vi "Get Column Headers.vi"(8 "error in (no error)":errorcluster, 11 "Process Tree View in":refnum<class "Process Tree View.lvclass">) -> (0 "error out":errorcluster, 3 "Process Tree View out":refnum<class "Process Tree View.lvclass">)   [LabVIEW 2020, in "Process Tree View.lvclass"]
uses:
  Process Tree View.lvclass
  Process Tree View.lvclass/Process Tree View.ctl
  Process Tree View Model/Process Tree View Model.lvclass
  Tree Helpers/Tag Tree/Tag Tree.lvclass
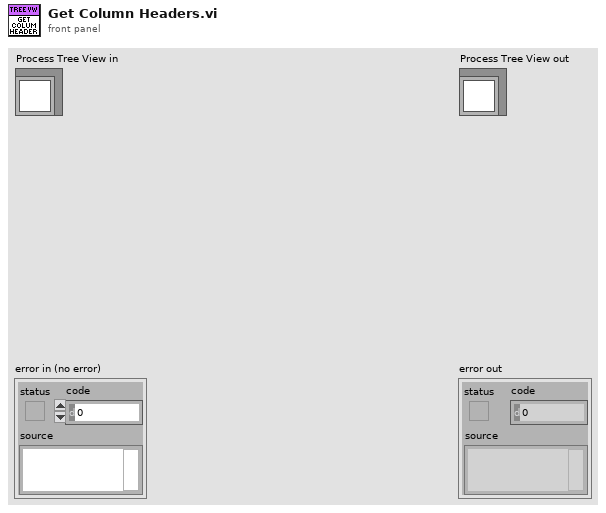
[diagram p1: front panel]
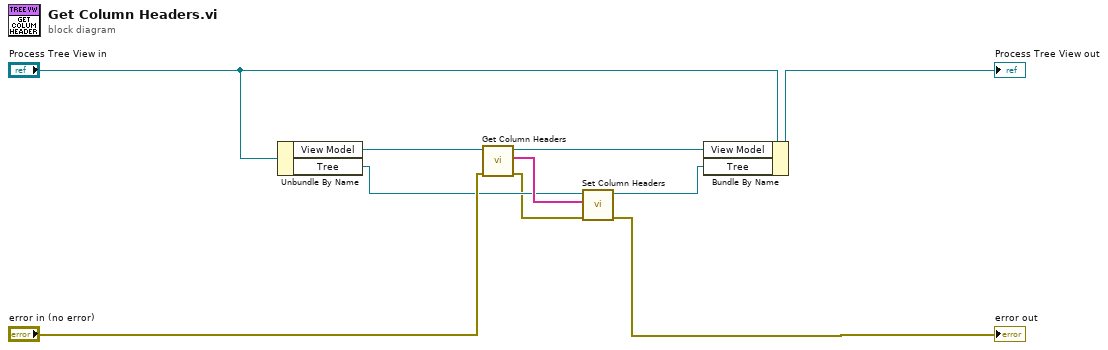
[diagram p0: block diagram]
diagram:
  n1 = Unbundle By Name("Process Tree View in") -> ("View Model"=w9:refnum<class "Process Tree View Model.lvclass">, "Tree"=w3:refnum<class "Tag Tree.lvclass">)
  n2 = call "Get Column Headers.vi"("error in (no error)"="error in (no error)", "List Box View Model in"=w9) -> ("error out"=w2:errorcluster, "Column Headers"=w5:string[], "List Box View Model out"=w6:refnum<class "Process Tree View Model.lvclass">)  [unwired: 7 in]
  n3 = call "Set Column Headers.vi"("error in (no error)"=w2, "Column Header Strings[]"=w5, "Tag Tree in"=w3) -> ("error out"=→"error out":errorcluster, "Tag Tree out"=w4:refnum<class "Tag Tree.lvclass">)  [unwired: 7 in]
  n4 = Bundle By Name(cluster="Process Tree View in", "View Model"=w6, "Tree"=w4) -> (→"Process Tree View out":refnum<class "Process Tree View.lvclass">)
